vi "Create Report Excel.vi"   [LabVIEW 2018, in "Application.lvlib"]
uses:
  Application.lvlib
  <vilib>/Utility/NIReport.llb/NI_report.lvclass
  <vilib>/Utility/NIReport.llb/Report Type.ctl
  <vilib>/Utility/NIReport.llb/NI_ReportGenerationCore.lvlib
  <vilib>/Utility/NIReport.llb/Append Text Table to Report (wrap).vi
types:
  T1 = typedef "NI_ReportGenerationCore.lvlib/Report Type.ctl" = enum16{"HTML", "Word", "Excel"}
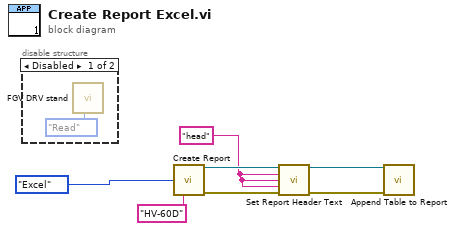
[diagram p0: block diagram]
diagram:
  w5 = "head" ("left header text")
  n1 = disable-structure shown="Disabled" {
    frame Disabled {
      n2 = call "FGV DRV stand.vi"("Enum"=enum16{"Write", "Read"}."Read") -> ()  [unwired: 10 in, 1 out]
    }
    frame Enabled {
    }
  }
  n3 = call <vilib>:"Create Report.vi"("report type"=Report_Type."Excel", "machine name (empty)"="HV-60D") -> ("report out"=w6:refnum<class "NI_report.lvclass">, "error out"=w4:errorcluster)  [unwired: 12 in]
  n4 = call-dynamic "Set Report Header Text.vi"("report in"=w6, "left header text"=w5, "center header text"=w5, "right header text"=w5, "error in (no error)"=w4) -> ("report out"=w3:refnum<class "NI_report.lvclass">, "error out"=w2:errorcluster)  [unwired: 9 in]
  n5 = call-poly <vilib>:"Append Table to Report.vi"("report in"=w3, "error in (no error)"=w2) -> ("column headers"=w1:string[])  [unwired: 9 in, 4 out]
